vi "6_Array Transform_solution.vi"(11 "Input Array":dbl[][](array[numeric])) -> (3 "Output Array":dbl[][](array[numeric]))   [LabVIEW 2014]
panel:
  # "Transfrom the input array into the output array \nsee the following example"
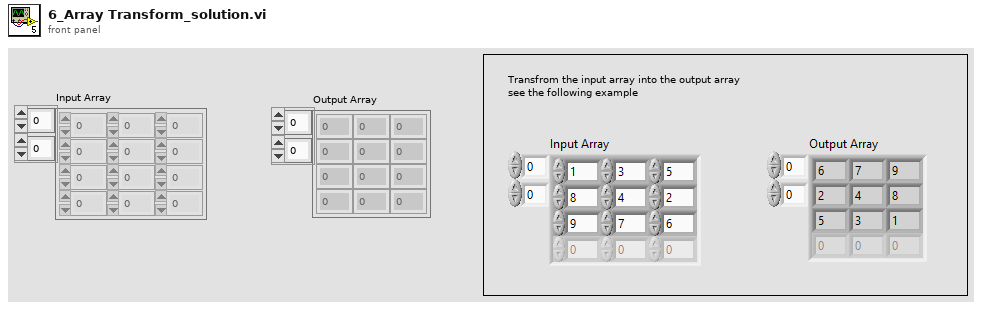
[diagram p1: front panel]
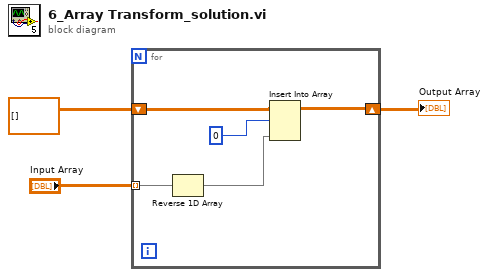
[diagram p0: block diagram]
diagram:
  n1 = for {
    tunnel: "Input Array" -> [w8] mode=indexing
    shift-right: [w5] -> w2
    shift-left: dbl[][] [] -> [w6]
    n2 = Reverse 1D Array(array=w8) -> (reversed array=w7:dbl[])
    n3 = Insert Into Array(array=w6, index (row)=0, new element=w7) -> (w5:dbl[][])  [unwired: 1 in]
  }
  "Output Array" <- w2
